vi "Read All Data.vi"(4 "Error In":errorcluster) -> (0 "Error Out":errorcluster, 3 "Ramp Data":dbl[](array[numeric]))   [LabVIEW 2015, in "Ramp Signal Data Buffer.lvlib"]
uses:
  Ramp Signal Data Buffer.lvlib
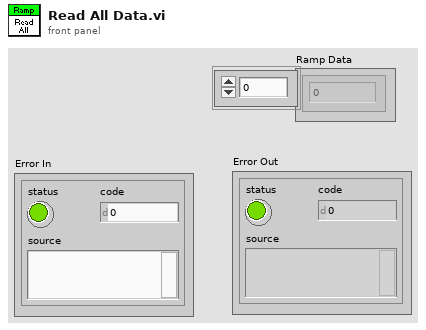
[diagram p1: front panel]
types:
  T1 = typedef "Ramp Signal Data Buffer.lvlib/buffer data typedef.ctl" = cluster{"Ramp Data":dbl[], "Counter":i32}
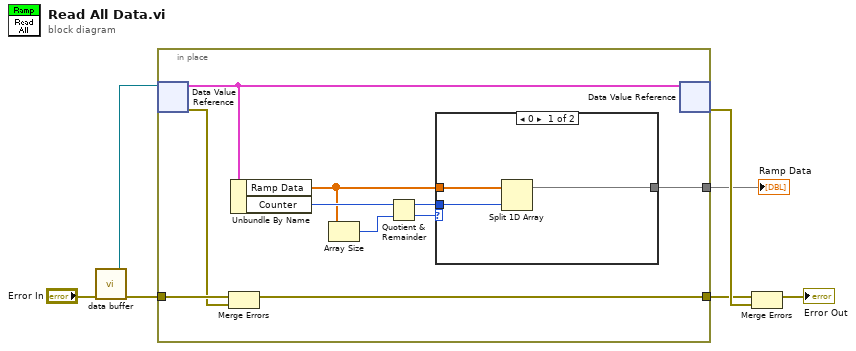
[diagram p0: block diagram]
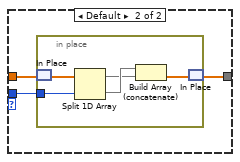
[diagram p2: hidden frame]
diagram:
  n1 = call "data buffer.vi"("Error In"="Error In") -> ("Error Out"=w2:errorcluster, "DVR"=w6:refnum<data-value>)  [unwired: 5 in]
  n2 = in-place {
    in-place-border: [w16] -> w3
    in-place-border: w2 -> [w15]
    in-place-border: [w13] -> w1
    n3 = in-place-dvr #1(w6) -> (w17:T1, w14:errorcluster)
    n4 = Merge Errors(w15, w14) -> (w13:errorcluster)
    n5 = Unbundle By Name(w17) -> ("Ramp Data"=w9:dbl[], "Counter"=w12:i32)
    n6 = Array Size(array=w9) -> (size(s)=w8:i32)
    n7 = Quotient & Remainder(x=w12, y=w8) -> (x-y*floor(x/y)=w10:i32, floor(x/y)=w11:i32)
    n8 = case shown="0" w11 {
      tunnel: w9 -> [w20 w23]
      tunnel: [w18 w22] -> w16
      tunnel: w10 -> [w19 w21]
      frame 0 {
        n9 = Split 1D Array(array=w20, index=w19) -> (first subarray=w18:dbl[])  [unwired: 1 out]
      }
      frame Default {
        n10 = in-place {
          in-place-border: w21 -> [w28]
          n11 = in-place-match #2(w23) -> (w25:dbl[])
          n12 = Split 1D Array(array=w25, index=w28) -> (first subarray=w26:dbl[], second subarray=w27:dbl[])
          n13 = Build Array (concatenate)(w27, w26) -> (w24:dbl[])
          n14 = in-place-match #2(w24) -> (w22:dbl[])
        }
      }
    }
    n15 = in-place-dvr #1(w17) -> (w7:errorcluster)  [unwired: 1 out]
  }
  "Ramp Data" <- w3
  n16 = Merge Errors(w1, w7) -> (→"Error Out":errorcluster)
